vi "Compare.vi"(8 "Image":T1, 9 "Cluster in":cluster{i32, i32, i32}, 10 "Image Pixels (U32) in":u32[][](array[numeric]), 11 "Image Pixels (U32) 3":u32[][](array[numeric])) -> (1 "Image Out":T1, 2 "Numeric":dbl, 3 "Image Pixels (U32) out":u32[][](array[numeric]))   [LabVIEW 2019]
uses:
  <vilib>/vision/Image Controls.llb/IMAQ Image.ctl
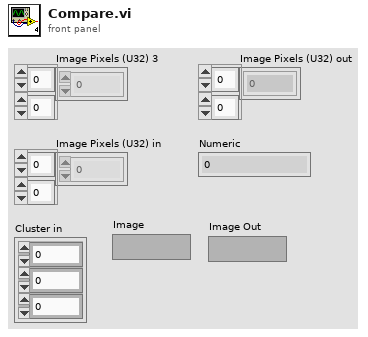
[diagram p1: front panel]
types:
  T1 = typedef "IMAQ Image.ctl" = refnum<image>
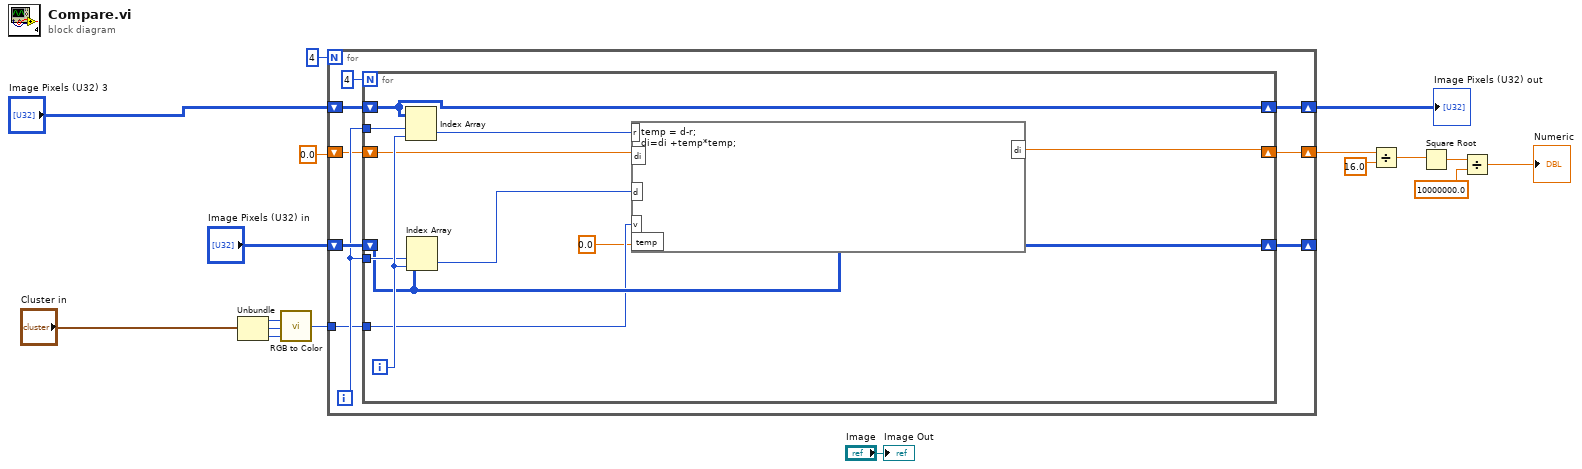
[diagram p0: block diagram]
diagram:
  n1 = Unbundle("Cluster in") -> (w13:i32, w14:i32, w15:i32)
  n2 = call <vilib>:"RGB to Color.vi"("B"=w15, "G"=w14, "R"=w13) -> ("Color"=w16:u32)
  n3 = for {
    N: 4 -> [_]
    shift-right: [w24] -> w10
    shift-left: "Image Pixels (U32) 3" -> [w25]
    shift-right: [w21] -> _
    shift-left: "Image Pixels (U32) in" -> [w23]
    tunnel: w16 -> [w20]
    shift-right: [w18] -> w6
    shift-left: 0.0 -> [w19]
    i -> [w22]
    n4 = for {
      N: 4 -> [_]
      shift-right: [w36] -> w24
      shift-left: w25 -> [w36]
      tunnel: w22 -> [w37]
      shift-right: [w33] -> w21
      shift-left: w23 -> [w33]
      tunnel: w22 -> [w34]
      tunnel: w20 -> [w32]
      shift-right: [w27] -> w18
      shift-left: w19 -> [w29]
      i -> [w35]
      n5 = Index Array(array=w36, index (row)=w37, index (col)=w35) -> (element=w31:u32)
      n6 = Index Array(array=w33, index (row)=w34, index (col)=w35) -> (element=w30:u32)
      n7 = formula code="temp = d-r;\ndi=di +temp*temp;"("v"=w32, "d"=w30, "r"=w31, "di"=w29, "temp"=0.0) -> ("di"=w27:dbl)
    }
  }
  "Image Pixels (U32) out" <- w10
  n8 = Divide(x=w6, y=16.0) -> (x/y=w4:dbl)
  n9 = Square Root(x=w4) -> (sqrt(x)=w3:dbl)
  n10 = Divide(x=w3, y=10000000.0) -> (x/y=→"Numeric":dbl)
  "Image Out" <- "Image"
